vi "CheesyDrive1712.vi"(6 "Quickturn":bool, 7 "SlowMode":u32=2, 10 "Wheel":dbl(slide) scale=-1.0..1.0, 11 "Throttle":dbl(slide)=-0.0 scale=-1.0..1.0) -> (2 "Right PWM":dbl=0.5949513901284444, 3 "Left PWM":dbl=0.5949513901284444)   [LabVIEW 2018]
doc: "Implements CheesyDrive. CheesyDrive means that the turn joystick controls the radius of turning instead of the rate of turning. Also implements QuickStop and QuickTurn."
panel:
  in  "FasterDeaccelerate":dbl=3.0
  in  "EnableHighSensRamp":dbl=0.8 format="%#_13g"
  in  "HighSensRamp":dbl=7.0 format="%#_13g"
  in  "ArrayOfSlownesss":T1(array[cluster])=[{"MaxSpeedSlow"=1.0, "SlowRate"=5.0, "MaxTurnSlow"=1.0, "MaxTurnRateSlow"=10.0}, {"MaxSpeedSlow"=0.6, "SlowRate"=4.0, "MaxTurnSlow"=0.8, "MaxTurnRateSlow"=10.0}, {"MaxSpeedSlow"=0.4, "SlowRate"=1.0, "MaxTurnSlow"=0.55, "MaxTurnRateSlow"=10.0}]
  in  "PointsTurn":cluster{"X":dbl, "Y":dbl}[](array[cluster])=[{"X"=0.0, "Y"=0.0}, {"X"=0.04, "Y"=0.0}, {"X"=0.041, "Y"=0.01}, {"X"=1.0, "Y"=1.0}, {"X"=1.0, "Y"=1.0}]
  in  "PointsQuickTurn":cluster{"X":dbl, "Y":dbl}[](array[cluster])=[{"X"=0.0, "Y"=0.0}, {"X"=0.04, "Y"=0.0}, {"X"=0.041, "Y"=0.2}, {"X"=0.9, "Y"=0.5}, {"X"=1.0, "Y"=1.0}]
  in  "PointsThrottle":cluster{"X":dbl, "Y":dbl}[](array[cluster])=[{"X"=0.0, "Y"=0.0}, {"X"=0.04, "Y"=0.0}, {"X"=0.0251, "Y"=0.15}, {"X"=1.0, "Y"=1.0}]
  in  "CarLikeTurning":bool
  in  "QSMult":dbl=0.1
  in  "WheelNonLinearity":dbl=0.65
  in  "negInertiaScalar":dbl=3.0
  in  "alpha":dbl=0.1
  out "Waveform Chart":dbl(graph)
  in  "Sensitivty":dbl=1.0
  # "Enable to enable"
  # "normal"
  # "(for quickstop decay)"
  # "Switch"
  # "Scale"
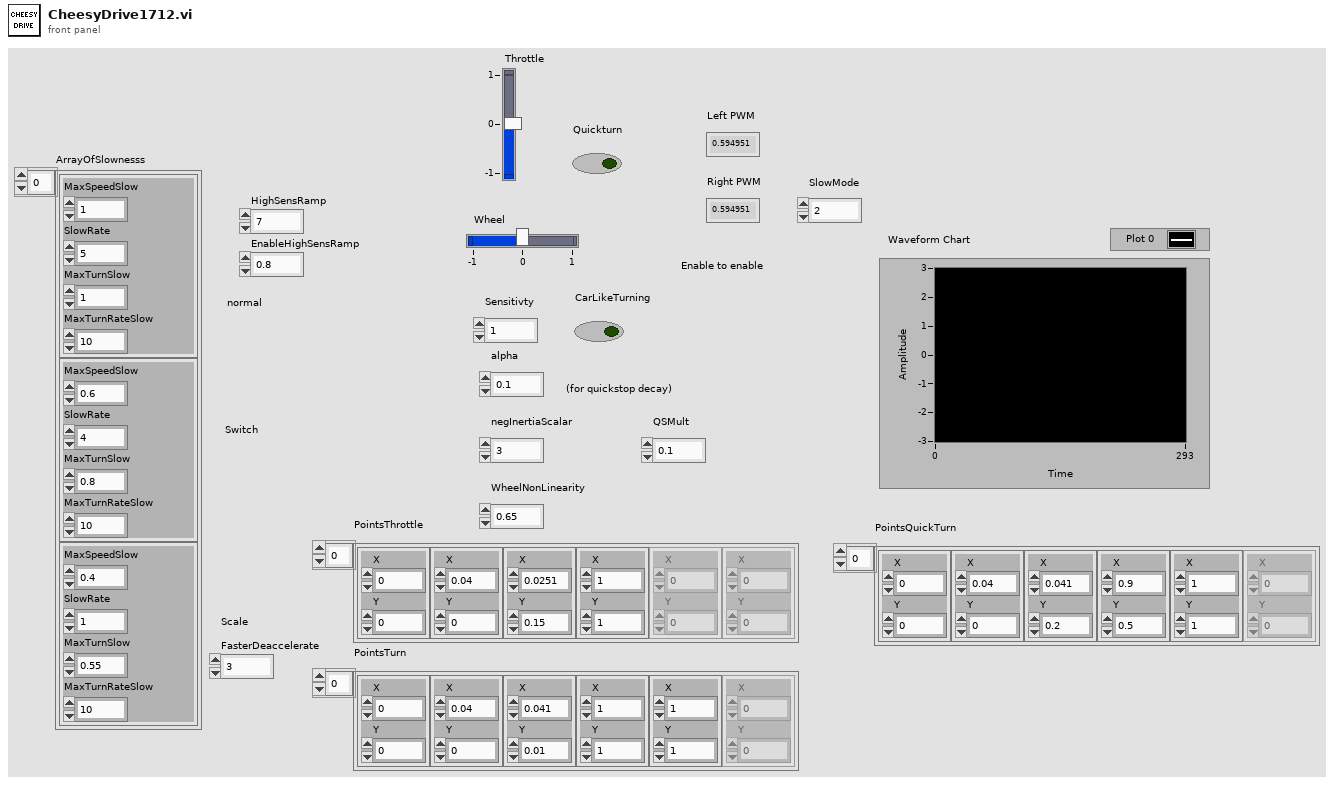
[diagram p1: front panel]
types:
  T1 = cluster{"MaxSpeedSlow":dbl, "SlowRate":dbl, "MaxTurnSlow":dbl, "MaxTurnRateSlow":dbl}[]
  T2 = cluster{"MaxSpeedSlow":dbl, "SlowRate":dbl, "MaxTurnSlow":dbl, "MaxTurnRateSlow":dbl}
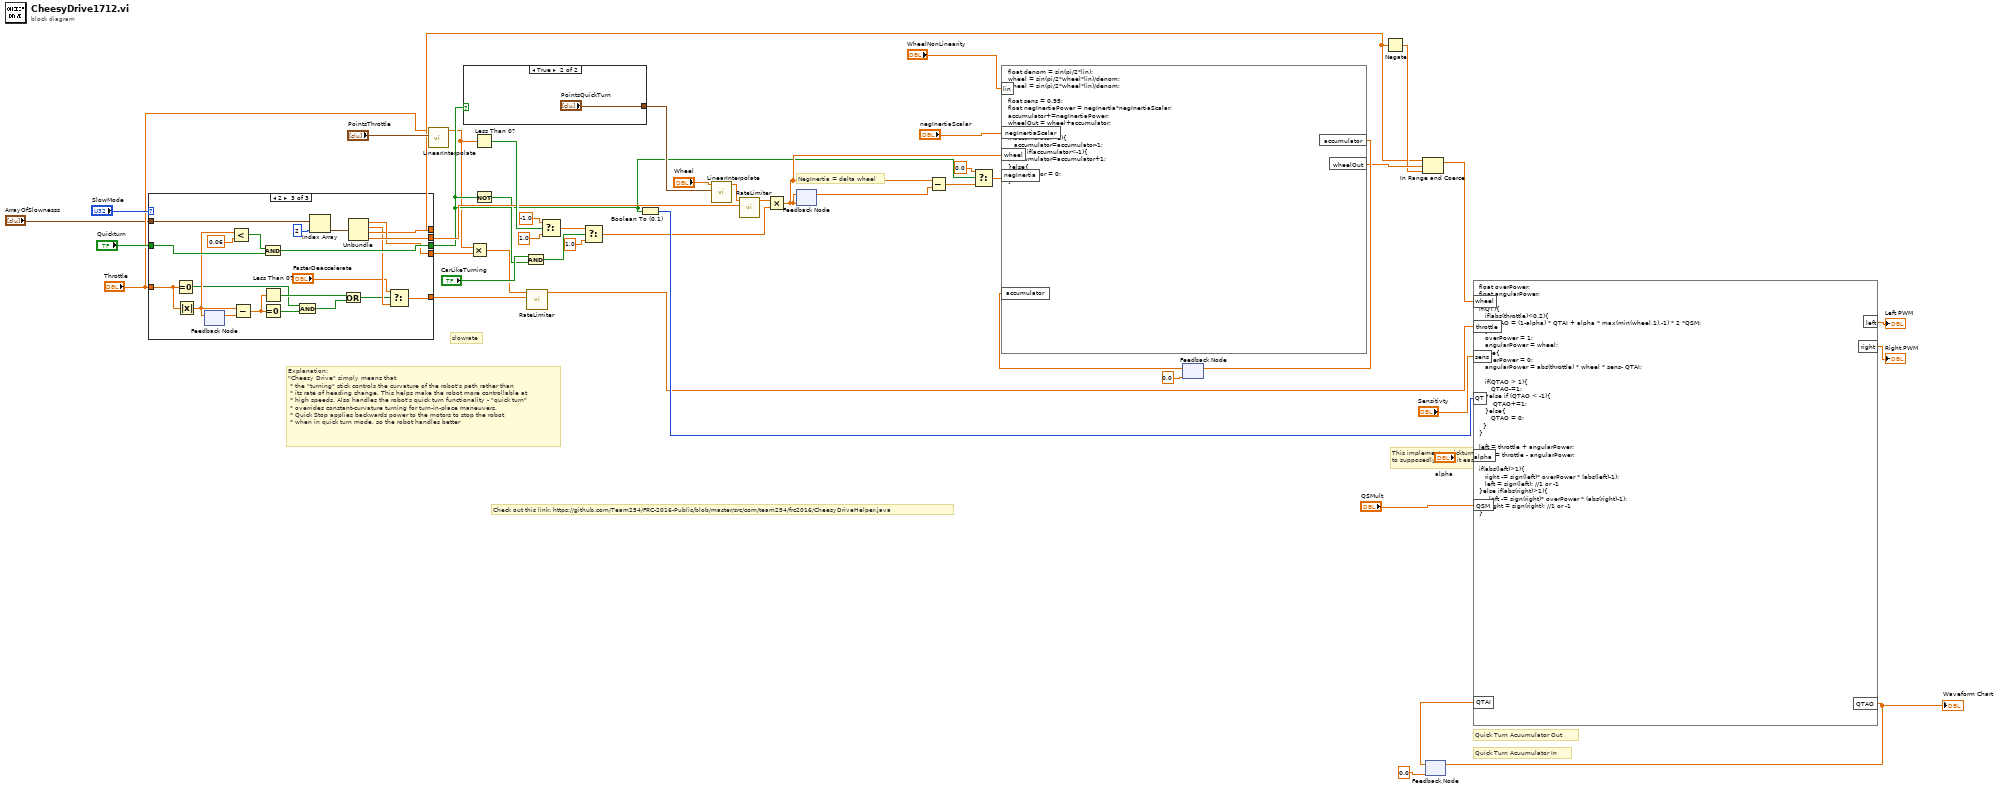
[diagram p0: block diagram]
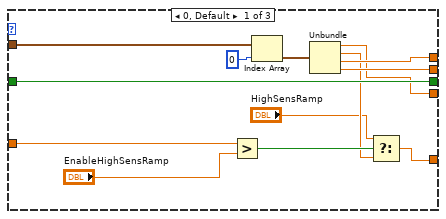
[diagram p2: hidden frame]
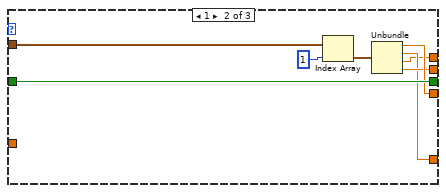
[diagram p3: hidden frame]
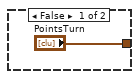
[diagram p4: hidden frame]
diagram:
  # "slowrate"
  # "This implements quickturn and also modifies wheel with a sine function\nto supposedly make it easier to drive"
  # "NegInertia = delta wheel"
  # "Explanation:\n\"Cheesy Drive\" simply means that\n * the \"turning\" stick controls the curvature of the robot's path rather than\n * its rate of heading change. This helps make the robot more controllable at\n * high speeds. Also handles the robot's quick turn functionality - \"quick turn\"\n * overrides constant-curvature turning for turn-in-place maneuvers.\n * Quick Stop applies backwards power to the motors to stop the robot\n * when in quick turn mode, so the robot handles better"
  # "Quick Turn Acuumulator Out"
  # "Quick Turn Acuumulator In"
  # "Check out this link: https://github.com/Team254/FRC-2016-Public/blob/master/src/com/team254/frc2016/CheesyDriveHelper.java"
  n1 = case shown="2" "SlowMode" {
    tunnel: [w49 w63 w78] -> w20
    tunnel: [w55 w65 w81] -> w2
    tunnel: [w56 w62 w80] -> w18
    tunnel: [w57 w64 w82] -> w15
    tunnel: "Quickturn" -> [w61 w69 w91]
    tunnel: [w61 w69 w88] -> w5
    tunnel: "Throttle" -> [w54 _ w75]
    tunnel: "ArrayOfSlownesss" -> [w58 w66 w85]
    frame 0, Default {
      n2 = Greater?(x=w54, y="EnableHighSensRamp") -> (0:w52:bool)
      n3 = Index Array(array=w58, index=0) -> (element=w59:T2)
      n4 = Unbundle(w59) -> ("MaxSpeedSlow"=w55:dbl, "SlowRate"=w51:dbl, "MaxTurnSlow"=w56:dbl, "MaxTurnRateSlow"=w57:dbl)
      n5 = Select(t="HighSensRamp", s=w52, f=w51) -> (s? t:f=w49:dbl)
    }
    frame 1 {
      n6 = Index Array(array=w66, index=1) -> (element=w67:T2)
      n7 = Unbundle(w67) -> ("MaxSpeedSlow"=w65:dbl, "SlowRate"=w63:dbl, "MaxTurnSlow"=w62:dbl, "MaxTurnRateSlow"=w64:dbl)
    }
    frame 2 {
      n8 = Equal To 0?(x=w75) -> (x = 0?=w74:bool)
      n9 = Absolute Value(x=w75) -> (abs(x)=w86:dbl)
      n10 = feedback-in #1(w86) -> ()
      n11 = feedback #1() -> (w87:dbl)  [unwired: 1 in]
      n12 = Less?(x=w86, y=0.06) -> (x < y?=w90:bool)
      n13 = Subtract(x=w86, y=w87) -> (x-y=w73:dbl)
      n14 = And(x=w90, y=w91) -> (x .and. y?=w88:bool)
      n15 = Less Than 0?(x=w73) -> (x < 0?=w76:bool)
      n16 = Equal To 0?(x=w73) -> (x = 0?=w71:bool)
      n17 = And(x=w74, y=w71) -> (x .and. y?=w72:bool)
      n18 = Index Array(array=w85, index=2) -> (element=w83:T2)
      n19 = Or(x=w76, y=w72) -> (x .or. y?=w70:bool)
      n20 = Unbundle(w83) -> ("MaxSpeedSlow"=w81:dbl, "SlowRate"=w79:dbl, "MaxTurnSlow"=w80:dbl, "MaxTurnRateSlow"=w82:dbl)
      n21 = Select(t="FasterDeaccelerate", s=w70, f=w79) -> (s? t:f=w78:dbl)
    }
  }
  n22 = call "LinearInterpolate.vi"("Points"="PointsThrottle", "Value"="Throttle") -> ("Output"=w4:dbl)  [unwired: 9 in]
  n23 = case shown="True" w5 {
    tunnel: ["PointsTurn" "PointsQuickTurn"] -> w22
    frame False {
    }
    frame True {
    }
  }
  n24 = Multiply(x=w4, y=w2) -> (x*y=w3:dbl)
  n25 = Less Than 0?(x=w4) -> (x < 0?=w30:bool)
  n26 = Not(x=w5) -> (.not. x?=w7:bool)
  n27 = And(x="CarLikeTurning", y=w7) -> (x .and. y?=w6:bool)
  n28 = call "RateLimiter.vi"("Max dx/dt"=w20, "Input"=w3) -> ("Output"=w42:dbl)  [unwired: 9 in]
  n29 = Select(t=-1.0, s=w30, f=1.0) -> (s? t:f=w26:dbl)
  n30 = Select(t=w26, s=w6, f=1.0) -> (s? t:f=w24:dbl)
  n31 = Boolean To (0,1)(Boolean=w5) -> (0, 1=w46:i16)
  n32 = call "LinearInterpolate.vi"("Points"=w22, "Value"="Wheel") -> ("Output"=w17:dbl)  [unwired: 9 in]
  n33 = call "RateLimiter.vi"("Max dx/dt"=w15, "Input"=w17) -> ("Output"=w16:dbl)  [unwired: 9 in]
  n34 = Multiply(x=w16, y=w24) -> (x*y=w27:dbl)
  n35 = feedback #2(w27) -> (w39:dbl)
  n36 = feedback-in #2(w27) -> ()
  n37 = Subtract(x=w27, y=w39) -> (x-y=w13:dbl)
  n38 = Select(t=0.0, s=w5, f=w13) -> (s? t:f=w14:dbl)
  n39 = feedback #3(0.0 ("Wheel")) -> (w38:dbl)
  n40 = formula code="float denom = sin(pi/2*lin);\nwheel = sin(pi/2*wheel*lin)/denom;\nwheel = sin(pi/2*wheel*lin)/denom;\n\nfloat sens = 0.95;\nfloat negInertiaPower = negInertia*negInertiaScalar;\naccumulator+=negInertiaPower;\nwheelOut = wheel+accumulator;\n\nif(accumulator>1){\n   accumulator=accumulator-1;\n}else if(accumulator<-1){\n   accumulator=accumulator+1;\n}else{\naccumulator = 0;\n}"("wheel"=w27, "negInertia"=w14, "accumulator"=w38, "negInertiaScalar"="negInertiaScalar", "lin"="WheelNonLinearity") -> ("accumulator"=w36:dbl, "wheelOut"=w32:dbl)
  n41 = feedback-in #3(w36) -> ()
  n42 = Negate(x=w18) -> (-x=w19:dbl)
  n43 = In Range and Coerce(upper limit=w18, x=w32, lower limit=w19) -> (coerced(x)=w33:dbl)  [unwired: 1 out]
  n44 = feedback #4(0.0 ("QTAccumulatorO")) -> (w44:dbl)
  n45 = formula code="float overPower;\nfloat angularPower;\n\nif(QT){\n   if(abs(throttle)<0.2){\n      QTAO = (1-alpha) * QTAI + alpha * max(min(wheel,1),-1) * 2 *QSM;\n   }\n   overPower = 1;\n   angularPower = wheel;\n}else{\n   overPower = 0;\n   angularPower = abs(throttle) * wheel * sens- QTAI;\n\n   if(QTAO > 1){\n      QTAO-=1;\n   }else if (QTAO < -1){\n       QTAO+=1;\n   }else{\n      QTAO = 0;\n  }\n}\n\nleft = throttle + angularPower;\nright = throttle - angularPower;\n\nif(abs(left)>1){\n   right -= sign(left)* overPower * (abs(left)-1);\n   left = sign(left); //1 or -1\n}else if(abs(right)>1){\n     left -= sign(right)* overPower * (abs(right)-1);\n     right = sign(right); //1 or -1 \n}"("wheel"=w33, "throttle"=w42, "sens"="Sensitivty", "QT"=w46, "alpha"="alpha", "QTAI"=w44, "QSM"="QSMult") -> ("left"=→"Left PWM":dbl, "right"=→"Right PWM":dbl, "QTAO"=w47:dbl)
  "Waveform Chart" <- w47
  n46 = feedback-in #4(w47) -> ()
